vi "TCP-Com_StandAlone.vi"(8 "Exit Control Label":string="Exit Button", 9 "pwd":string, 10 "LabView Port":u16=4000, 11 "VI Refnum":refnum<vi>) -> (0 "error out":errorcluster)   [LabVIEW 2019]
doc: "This template is for the Queued Message Handler design pattern.\n\nThe Event Handling Loop generates messages based on user interface actions.\n\nThe Message Handling Loop processes messages generated by the Event Handling Loop, or by other messages. The messages are string values, so new messages can be added easily to the Message Cases case structure in the Message Handling Loop. Each message cluster can also provide an optional value for Message Data, which is a variant that can be converted to whatever message-specific data is required."
uses:
  support/TPC-Enum.ctl
  support/Global 1.vi
  support/Message Queue/Enqueue Message (Single).vi
  <vilib>/Utility/error.llb/Error Cluster From Error Code.vi
  <vilib>/ErrorRing/Error Ring.xnode
  support/Message Queue/Message Queue.lvlib
  support/User Event - Stop/User Event - Stop.lvlib
panel:
  out "Try reques  Bool":bool
  out "Sent to MIDAS":string
  out "connection ID":refnum<k5>
  out "Client Connected":bool
  in  "Request":string
  in  "Try request":bool
  in  "Exit":bool
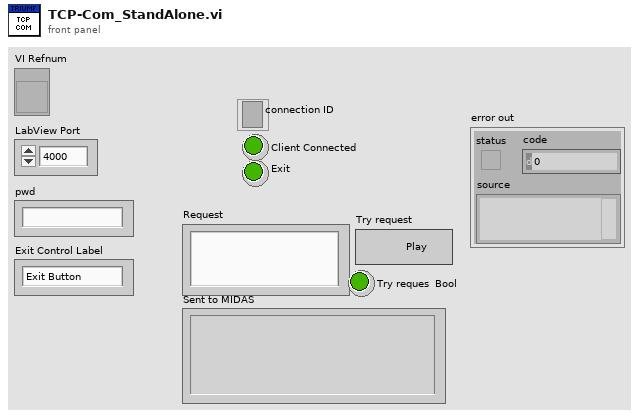
[diagram p1: front panel]
types:
  T1 = typedef "TPC-Enum.ctl" = enum16{"Wait For Client", "Check Client", "Listen"}
  T2 = typedef "Message Queue.lvlib/All Message Queues.ctl" = cluster{"TCP":refnum<queue>}
  T3 = enum16{"Standard", "Buffered", "CRLF", "Immediate"}
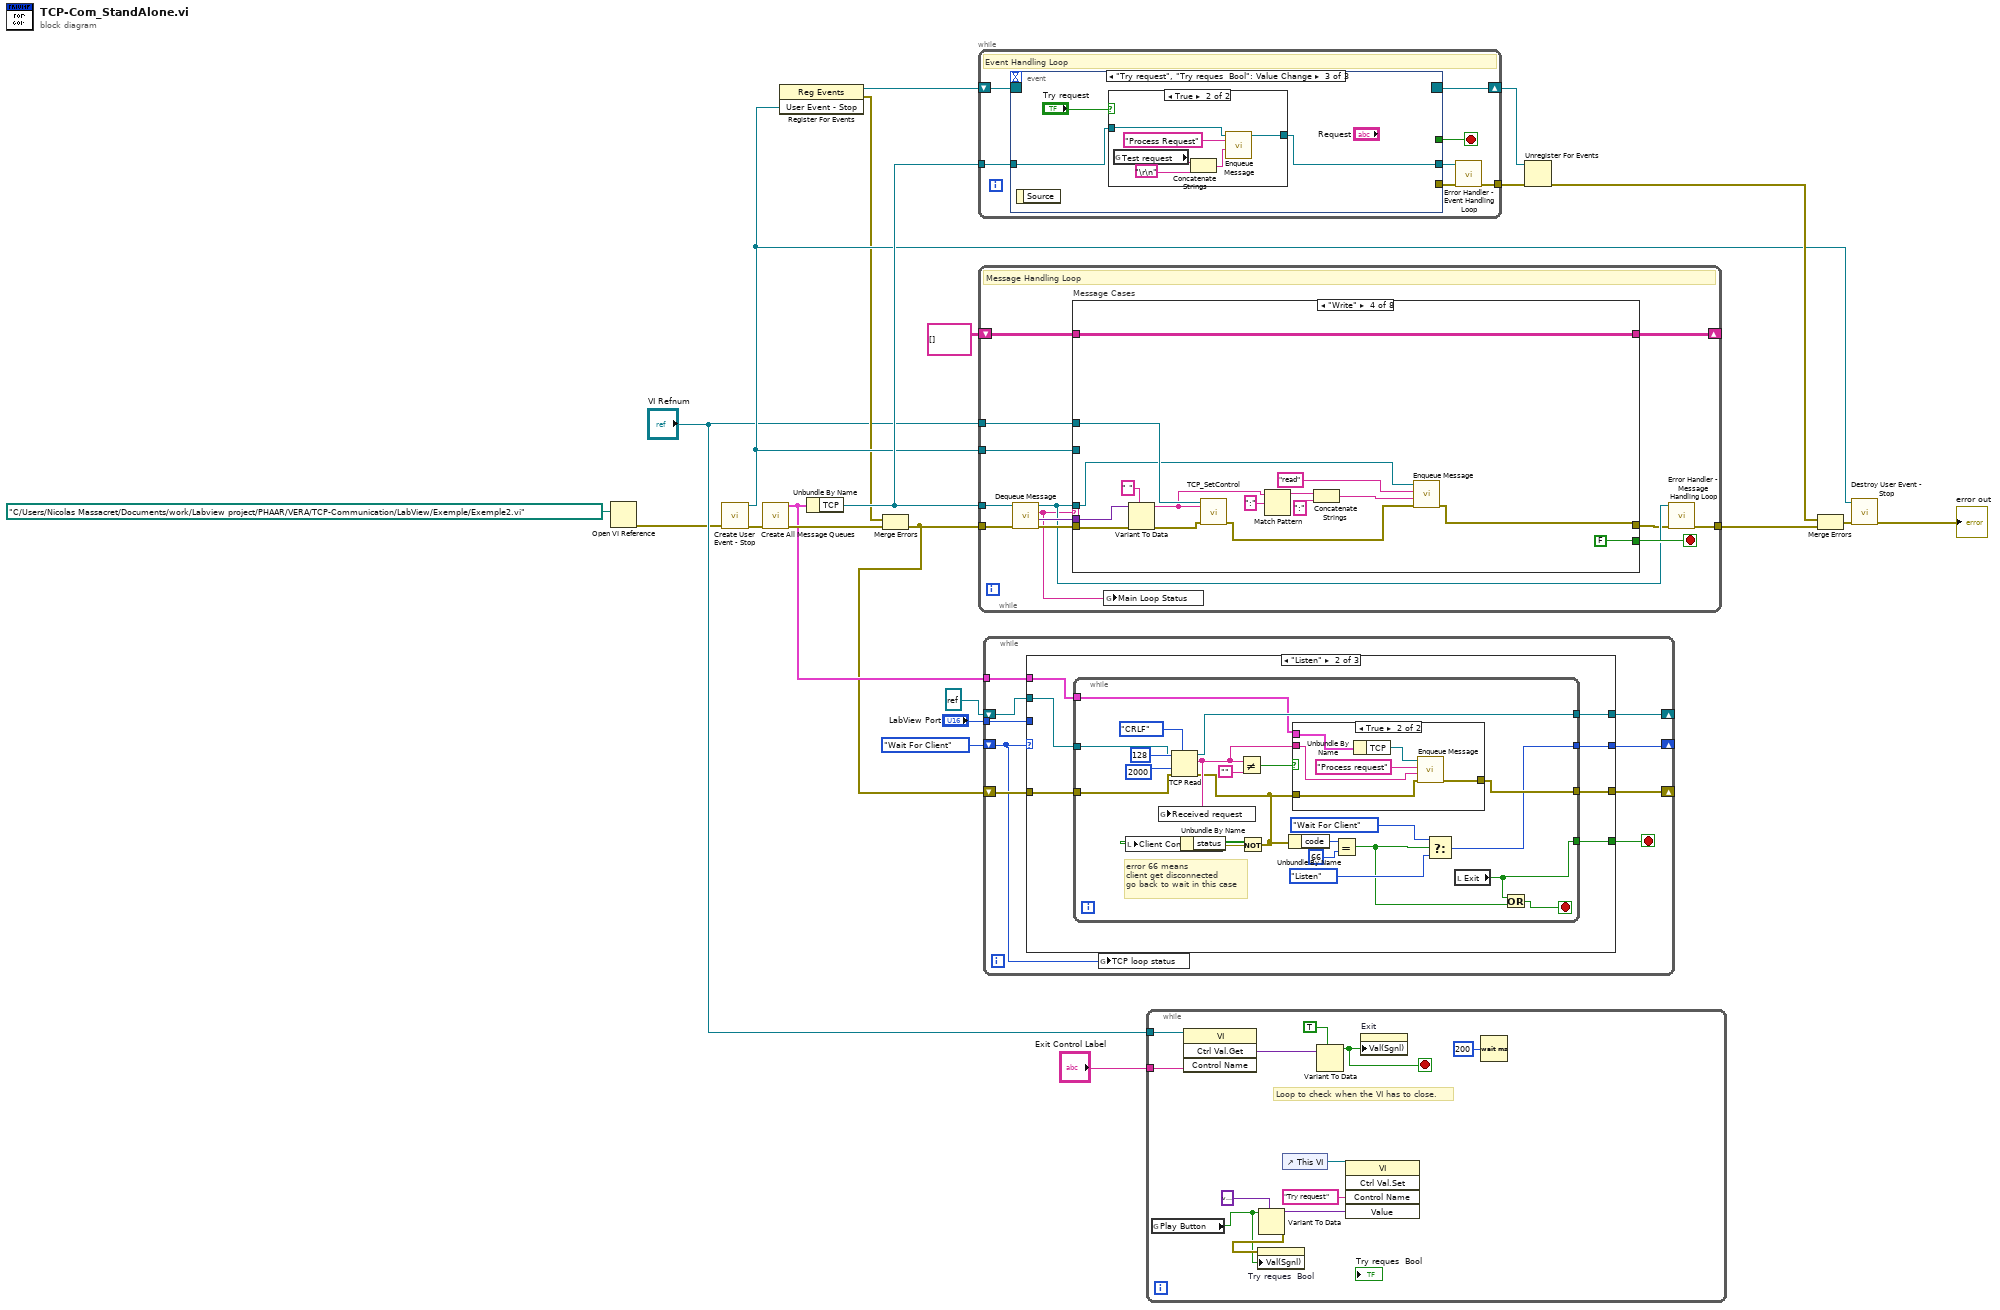
[diagram p0: block diagram]
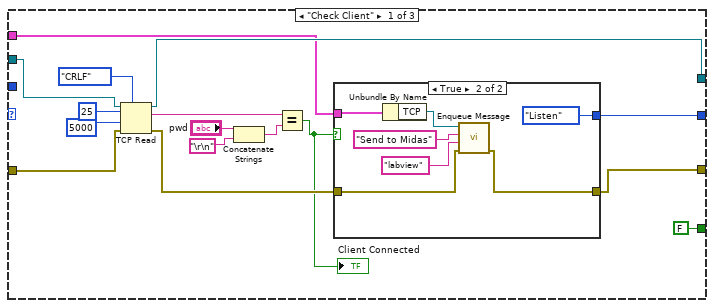
[diagram p2: hidden frame]
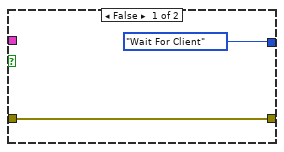
[diagram p3: hidden frame]
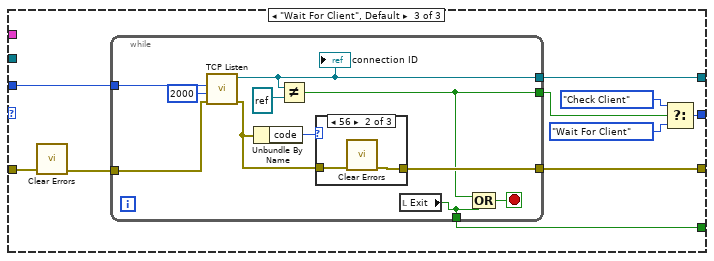
[diagram p5: hidden frame]
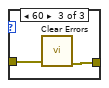
[diagram p7: hidden frame]
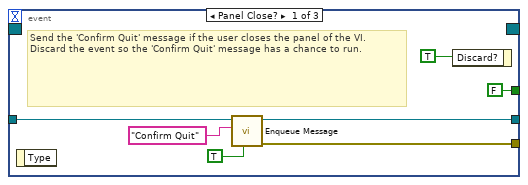
[diagram p8: hidden frame]
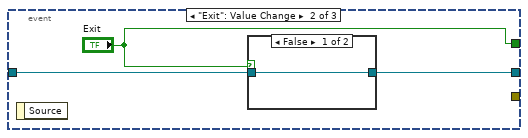
[diagram p9: hidden frame]
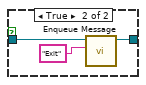
[diagram p10: hidden frame]
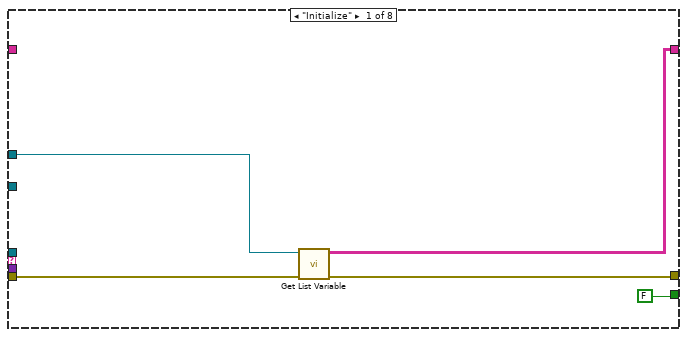
[diagram p12: hidden frame]
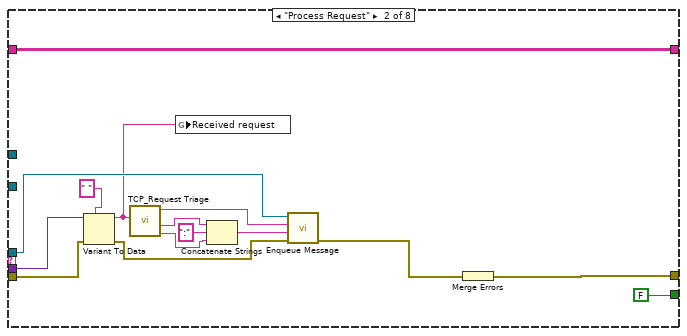
[diagram p13: hidden frame]
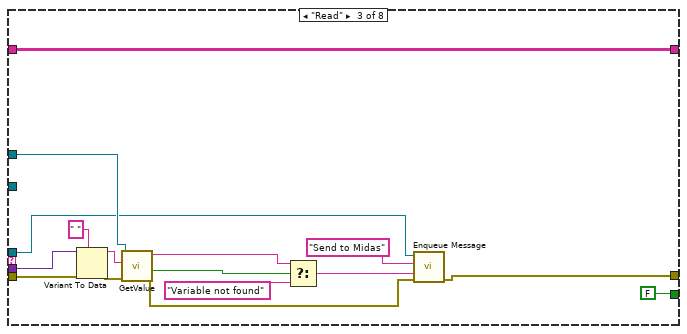
[diagram p14: hidden frame]
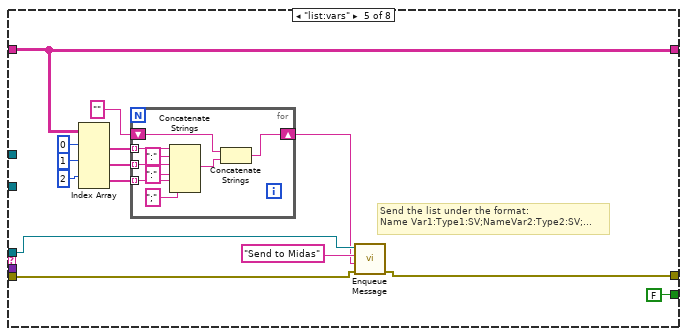
[diagram p15: hidden frame]
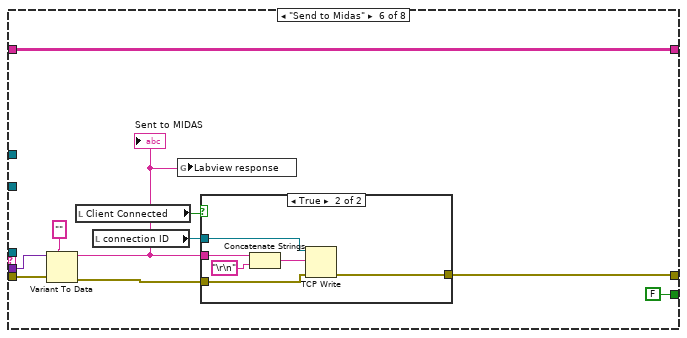
[diagram p16: hidden frame]
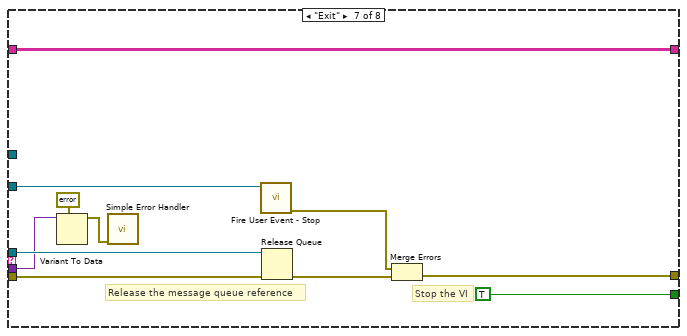
[diagram p18: hidden frame]
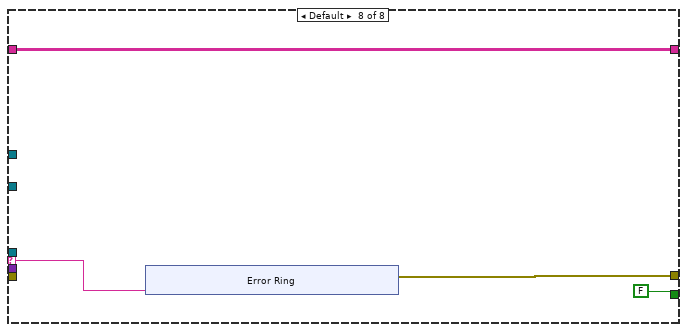
[diagram p19: hidden frame]
diagram:
  n1 = Open VI Reference(vi path=path "C:/Users/Nicolas Massacret/Documents/work/Labview project/PHAAR/VERA/TCP-Communication/LabView/Exemple/Exemple2.vi") -> (error out=w2:errorcluster)  [unwired: 5 in, 1 out]
  n2 = call "Create User Event - Stop.vi"("error in (no error)"=w2) -> ("error out"=w19:errorcluster, "User Event - Stop"=w13:refnum<user-event>)  [unwired: 9 in]
  n3 = call "Create All Message Queues.vi"("error in (no error)"=w19) -> ("error out"=w22:errorcluster, "Message Queues out"=w8:T2)  [unwired: 9 in]
  n4 = register-events(w13) -> (reference out=w14:refnum<event-registration>, error out=w12:errorcluster)  [unwired: 2 in]
  n5 = Unbundle By Name(w8) -> ("TCP"=w20:refnum<queue>)
  n6 = Merge Errors(w12, w22) -> (w4:errorcluster)
  n7 = while {
    tunnel: w20 -> [w29]
    shift-right: [w27] -> w16
    shift-left: w14 -> [w28]
    tunnel: [w23] -> w15
    stop <- w25 stop-if-true
    # "Event Handling Loop"
    n8 = event shown="[2] \"Try request\", \"Try reques  Bool\": Value Change" {
      selector: w28 -> [_ _ _]
      dyn-events: [_ _ _] -> w27
      timeout: _ -> [_ _ _]
      tunnel: [FALSE ("Discard?") "Exit" _] -> w25
      tunnel: w29 -> [w35 w39 w45]
      tunnel: [w34 _ _] -> w26
      tunnel: [w33 w38 w44] -> w24
      event Panel Close? {
        # "Send the 'Confirm Quit' message if the user closes the panel of the VI. Discard the event so the 'Confirm Quit' message has a chance to run."
        n9 = event-data() -> ()  [unwired: 1 in, 1 out]
        n10 = call-poly "Enqueue Message.vi"("Priority Message? (F)"=TRUE, "Message"="Confirm Quit", "Message Queue"=w35) -> ("error out"=w34:errorcluster, "dup Message Queue"=w33:refnum<queue>)  [unwired: 7 in]
        n11 = event-data("Discard?"=TRUE) -> ()  [unwired: 1 in, 1 out]
      }
      event "Exit": Value Change {
        n12 = event-data() -> ()  [unwired: 1 in, 1 out]
        n13 = case shown="False" "Exit" {
          tunnel: w39 -> [w40 w43]
          tunnel: [w40 w41] -> w38
          frame False {
          }
          frame True {
            n14 = call-poly "Enqueue Message.vi"("Message"="Exit", "Message Queue"=w43) -> ("dup Message Queue"=w41:refnum<queue>)  [unwired: 8 in, 1 out]
          }
        }
      }
      event "Try request", "Try reques  Bool": Value Change {
        n15 = event-data() -> ()  [unwired: 1 in, 1 out]
        n16 = case shown="True" "Try request" {
          tunnel: w45 -> [w47 w53]
          tunnel: [w47 w52] -> w44
          frame False {
          }
          frame True {
            n17 = global read "Global 1.vi" "Test request"() -> (w48:string)
            n18 = Concatenate Strings(w48, "\r\n") -> (w51:string)
            n19 = call-poly "Enqueue Message.vi"("Message Data"=w51, "Message"="Process Request", "Message Queue"=w53) -> ("dup Message Queue"=w52:refnum<queue>)  [unwired: 7 in, 1 out]
          }
        }
      }
    }
    n20 = call "Error Handler - Event Handling Loop.vi"("error in (no error)"=w26, "Message Queue"=w24) -> ("dup error in"=w23:errorcluster)  [unwired: 8 in, 1 out]
  }
  n21 = while {
    tunnel: w20 -> [w61]
    tunnel: w13 -> [w65]
    tunnel: w4 -> [w64]
    tunnel: [w59] -> w21
    tunnel: "VI Refnum" -> [w57]
    shift-right: [w56] -> _
    shift-left: string[][] [] -> [w55]
    stop <- w66 stop-if-true
    # "Message Handling Loop"
    n22 = call "Dequeue Message.vi"("error in (no error)"=w64, "Message Queue"=w61) -> ("error out"=w63:errorcluster, "Message Data"=w62:variant, "Message"=w54:string, "dup Message Queue"=w60:refnum<queue>)  [unwired: 6 in]
    n23 = case "Message Cases" shown="\"Write\"" w54 {
      selector: w54 -> [_ _ _ _ _ _ _ w172]
      tunnel: w60 -> [_ w79 w88 w105 w131 _ w169 _]
      tunnel: w63 -> [w70 w84 w101 w117 w130 w149 w163 _]
      tunnel: [w67 w86 w87 w103 w129 w143 w166 w173] -> w58
      tunnel: [FALSE FALSE FALSE FALSE FALSE FALSE TRUE FALSE] -> w66
      tunnel: w62 -> [_ w85 w102 w116 _ w148 w160 _]
      tunnel: w65 -> [_ _ _ _ _ _ w165 _]
      tunnel: w57 -> [w69 _ w95 w113 _ _ _ _]
      tunnel: [w68 w73 w98 w114 w127 w151 w159 w170] -> w56
      tunnel: w55 -> [_ w73 w98 w114 w127 w151 w159 w170]
      frame "Initialize" {
        # "Initialize - All initialization work should take place in this message, since other loops can potentially enqueue messages that execute immediately after this one."
        n24 = call "Get List Variable.vi"("error in (no error)"=w70, "VI in"=w69) -> ("error out"=w67:errorcluster, "Array"=w68:string[][])  [unwired: 8 in]
      }
      frame "Process Request" {
        # "Something - Replace this message with functionality for your own application."
        n25 = Variant To Data(error in=w84, type=" " ("Message"), Variant=w85) -> (data=w72:string, error out=w80:errorcluster)
        n26 = call "TCP_Request Triage.vi"("Message"=w72) -> ("Value"=w75:string, "Variable"=w76:string, "Request"=w77:string)  [unwired: 8 in]
        n27 = global write "Global 1.vi" "Received request"(w72) -> ()
        n28 = Concatenate Strings(w76, ":" ("string"), w75) -> (w78:string)
        n29 = call-poly "Enqueue Message.vi"("error in (no error)"=w80, "Message Data"=w78, "Message"=w77, "Message Queue"=w79) -> ("error out"=w81:errorcluster)  [unwired: 6 in, 1 out]
        n30 = Merge Errors(w81) -> (w86:errorcluster)
      }
      frame "Read" {
        n31 = Variant To Data(error in=w101, type=" " ("Message"), Variant=w102) -> (data=w96:string, error out=w97:errorcluster)
        n32 = call "GetValue.vi"("reference"=w95, "Input"=w96, "error in (no error)"=w97) -> ("Answer"=w92:string, "Found?"=w93:bool, "error out"=w91:errorcluster)  [unwired: 5 in]
        n33 = Select(t=w92, s=w93, f="Variable not found") -> (s? t:f=w89:string)
        n34 = call-poly "Enqueue Message.vi"("error in (no error)"=w91, "Message Data"=w89, "Message"="Send to Midas", "Message Queue"=w88) -> ("error out"=w87:errorcluster)  [unwired: 6 in, 1 out]
      }
      frame "Write" {
        n35 = Variant To Data(error in=w117, type=" " ("Message"), Variant=w116) -> (data=w108:string, error out=w112:errorcluster)
        n36 = call "TCP_SetControl.vi"("VI Refnum"=w113, "Input"=w108, "error in (no error)"=w112) -> ("error out"=w104:errorcluster)  [unwired: 6 in, 1 out]
        n37 = Match Pattern(string=w108, regular expression=":") -> (before substring=w106:string)  [unwired: 1 in, 3 out]
        n38 = Concatenate Strings(w106, ":" ("string")) -> (w110:string)
        n39 = call-poly "Enqueue Message.vi"("error in (no error)"=w104, "Message Data"=w110, "Message"="read", "Message Queue"=w105) -> ("error out"=w103:errorcluster)  [unwired: 6 in, 1 out]
      }
      frame "list:vars" {
        # "Send the list under the format:\nName Var1:Type1:SV;NameVar2:Type2:SV;..."
        n40 = Index Array(array=w127, index (row) #1=0 ("index (row)"), index (row) #2=1 ("index (row)"), index (row) #3=2 ("index (row)")) -> (element #1=w125:string[], element #2=w123:string[], element #3=w119:string[])  [unwired: 3 in]
        n41 = for {
          tunnel: w125 -> [w141] mode=indexing
          tunnel: w123 -> [w139] mode=indexing
          shift-right: [w135] -> w121
          shift-left: "" -> [w137]
          tunnel: w119 -> [w134] mode=indexing
          n42 = Concatenate Strings(w141, ":" ("string"), w139, ":" ("string"), w134, ";" ("string")) -> (w136:string)
          n43 = Concatenate Strings(w137, w136) -> (w135:string)
        }
        n44 = call-poly "Enqueue Message.vi"("error in (no error)"=w130, "Message Data"=w121, "Message"="Send to Midas", "Message Queue"=w131) -> ("error out"=w129:errorcluster)  [unwired: 6 in, 1 out]
      }
      frame "Send to Midas" {
        n45 = Variant To Data(error in=w149, type="", Variant=w148) -> (data=w142:string, error out=w144:errorcluster)
        "Sent to MIDAS" <- w142
        n46 = local read "Client Connected"() -> (w146:bool)
        n47 = local read "connection ID"() -> (w145:refnum<k5>)
        n48 = global write "Global 1.vi" "Labview response"(w142) -> ()
        n49 = case shown="True" w146 {
          tunnel: w145 -> [_ w155]
          tunnel: w142 -> [_ w158]
          tunnel: w144 -> [w152 w156]
          tunnel: [w152 w154] -> w143
          frame False {
          }
          frame True {
            n50 = Concatenate Strings(w158, "\r\n") -> (w153:string)
            n51 = TCP Write(connection ID=w155, data in=w153, error in (no error)=w156) -> (error out=w154:errorcluster)  [unwired: 1 in, 2 out]
          }
        }
      }
      frame "Exit" {
        # "Stop the VI"
        # "Release the message queue reference"
        # "Exit - Exit the application."
        n52 = Variant To Data(type=errorcluster {"status"=FALSE, "code"=0, "source"=""} ("error constant"), Variant=w160) -> (data=w161:errorcluster)  [unwired: 1 in, 1 out]
        n53 = call <vilib>:"Simple Error Handler.vi"("error in (no error)"=w161) -> ()  [unwired: 4 in, 5 out]
        n54 = call "Fire User Event - Stop.vi"("User Event - Stop"=w165) -> ("error out"=w164:errorcluster)  [unwired: 10 in]
        n55 = Release Queue(queue=w169, error in (no error)=w163) -> (error out=w167:errorcluster)  [unwired: 1 in, 2 out]
        n56 = Merge Errors(w164, w167) -> (w166:errorcluster)
      }
      frame Default {
        # "'Default' case only runs if there is a message that isn't defined in any of the other cases.  Output a programming error."
        n57 = xnode "Error Ring"("parameter 0"=w172) -> ("error out"=w173:errorcluster)
      }
    }
    n58 = global write "Global 1.vi" "Main Loop Status"(w54) -> ()
    n59 = call "Error Handler - Message Handling Loop.vi"("error in (no error)"=w58, "Message Queue"=w60) -> ("dup error in"=w59:errorcluster)  [unwired: 8 in, 1 out]
  }
  n60 = while {
    shift-right: [w187] -> _
    shift-left: TPC-Enum."Wait For Client" -> [w181]
    tunnel: "LabView Port" -> [w189]
    shift-right: [w188] -> _
    shift-left: refnum<k5> refnum ("connection ID") -> [w183]
    shift-right: [w186] -> _
    shift-left: w4 -> [w185]
    tunnel: w8 -> [w182]
    stop <- w184 stop-if-true
    n61 = case shown="\"Listen\"" w181 {
      tunnel: w189 -> [_ _ w260]
      tunnel: w185 -> [w202 w220 w252]
      tunnel: [w196 w219 w259] -> w188
      tunnel: [w193 w216 w255] -> w187
      tunnel: [FALSE w215 w254] -> w184
      tunnel: [w192 w217 w253] -> w186
      tunnel: w183 -> [w201 w221 _]
      tunnel: w182 -> [w195 w218 _]
      frame "Check Client" {
        n62 = TCP Read(connection ID=w201, bytes to read=25, error in (no error)=w202, 7:T3."CRLF" ("mode (standard)"), 9:5000 ("timeout ms (25000)")) -> (connection ID out=w196:refnum<k5>, data out=w198:string, error out=w194:errorcluster)
        n63 = Concatenate Strings("pwd", "\r\n") -> (w197:string)
        n64 = Equal?(x=w198, y=w197) -> (x = y?=w190:bool)
        "Client Connected" <- w190
        n65 = case shown="True" w190 {
          tunnel: w195 -> [_ w214]
          tunnel: w194 -> [w207 w210]
          tunnel: [TPC-Enum."Wait For Client" TPC-Enum."Listen"] -> w193
          tunnel: [w207 w208] -> w192
          frame False {
          }
          frame True {
            n66 = Unbundle By Name(w214) -> ("TCP"=w213:refnum<queue>)
            n67 = call-poly "Enqueue Message.vi"("error in (no error)"=w210, "Message Data"="labview", "Message"="Send to Midas", "Message Queue"=w213) -> ("error out"=w208:errorcluster)  [unwired: 6 in, 1 out]
          }
        }
      }
      frame "Listen" {
        n68 = while {
          tunnel: w221 -> [w240]
          tunnel: w220 -> [w239]
          tunnel: [w236] -> w219
          tunnel: w218 -> [w235]
          tunnel: [w234] -> w217
          tunnel: [w230] -> w216
          tunnel: [w224] -> w215
          stop <- w223 stop-if-true
          # "error 66 means\nclient get disconnected\ngo back to wait in this case"
          n69 = TCP Read(connection ID=w240, bytes to read=128, error in (no error)=w239, 7:T3."CRLF" ("mode (standard)"), 9:2000 ("timeout ms (25000)")) -> (connection ID out=w236:refnum<k5>, data out=w228:string, error out=w227:errorcluster)
          n70 = global write "Global 1.vi" "Received request"(w228) -> ()
          n71 = Unbundle By Name(w227) -> ("status"=w233:bool)
          n72 = Not Equal?(x=w228, y="") -> (x != y?=w237:bool)
          n73 = Not(x=w233) -> (.not. x?=w229:bool)
          n74 = local write "Client Connected"(w229) -> ()
          n75 = Unbundle By Name(w227) -> ("code"=w226:i32)
          n76 = case shown="True" w237 {
            tunnel: w228 -> [_ w247]
            tunnel: w235 -> [_ w248]
            tunnel: w227 -> [w244 w246]
            tunnel: [w244 w245] -> w234
            frame False {
            }
            frame True {
              n77 = Unbundle By Name(w248) -> ("TCP"=w250:refnum<queue>)
              n78 = call-poly "Enqueue Message.vi"("error in (no error)"=w246, "Message Data"=w247, "Message"="Process request", "Message Queue"=w250) -> ("error out"=w245:errorcluster)  [unwired: 6 in, 1 out]
            }
          }
          n79 = Equal?(x=w226, y=66) -> (x = y?=w222:bool)
          n80 = Select(t=TPC-Enum."Wait For Client", s=w222, f=TPC-Enum."Listen") -> (s? t:f=w230:T1)
          n81 = local read "Exit"() -> (w224:bool)
          n82 = Or(x=w224, y=w222) -> (x .or. y?=w223:bool)
        }
      }
      frame "Wait For Client", Default {
        n83 = call <vilib>:"Clear Errors.vi"("error in (no error)"=w252) -> ("error out"=w251:errorcluster)  [unwired: 5 in, 1 out]
        n84 = while {
          tunnel: w260 -> [w271]
          tunnel: w251 -> [w269]
          tunnel: [w262] -> w258
          tunnel: [w267] -> w259
          tunnel: [w264] -> w253
          tunnel: [w261] -> w254
          stop <- w263 stop-if-true
          n85 = call <vilib>:"TCP Listen.vi"("error in (no error)"=w269, "timeout ms (wait forever: -1)"=2000, "port"=w271) -> ("error out"=w265:errorcluster, "connection ID"=w267:refnum<k5>)  [unwired: 4 in, 3 out]
          "connection ID" <- w267
          n86 = Unbundle By Name(w265) -> ("code"=w266:i32)
          n87 = Not Equal?(x=w267, y=refnum<k5> refnum ("connection ID")) -> (x != y?=w262:bool)
          n88 = case shown="56" w266 {
            tunnel: w265 -> [w272 w274 w276]
            tunnel: [w272 w273 w275] -> w264
            frame 0, Default {
            }
            frame 56 {
              n89 = call <vilib>:"Clear Errors.vi"("error in (no error)"=w274) -> ("error out"=w273:errorcluster)  [unwired: 5 in, 1 out]
            }
            frame 60 {
              n90 = call <vilib>:"Clear Errors.vi"("error in (no error)"=w276) -> ("error out"=w275:errorcluster)  [unwired: 5 in, 1 out]
            }
          }
          n91 = local read "Exit"() -> (w261:bool)
          n92 = Compound Arithmetic op=OR(w262, w261) -> (w263:bool)
        }
        n93 = Select(t=TPC-Enum."Check Client", s=w258, f=TPC-Enum."Wait For Client") -> (s? t:f=w255:T1)
      }
    }
    n94 = global write "Global 1.vi" "TCP loop status"(w181) -> ()
  }
  n95 = while {
    tunnel: "VI Refnum" -> [w283]
    tunnel: "Exit Control Label" -> [w284]
    stop <- w286 stop-if-true
    # "Loop to check when the VI has to close."
    n96 = global read "Global 1.vi" "Play Button"() -> (w277:bool)
    n97 = invoke class="VI" method="Ctrl Val.Get"(reference=w283, "Control Name"=w284) -> ("Get Control Value Variant"=w285:variant)  [unwired: 2 in, 3 out]
    n98 = Variant To Data(type=variant ("Value (Signaling)"), Variant=w277) -> (data=w280:variant, error out=w278:errorcluster)  [unwired: 1 in]
    n99 = property on="Try reques  Bool" class="Bool (strict)"(error in=w278, "Val(Sgnl)"=w277) -> ()  [unwired: 1 in, 2 out]
    n100 = control-ref of="This VI"() -> (w281:refnum<vi>)
    n101 = Variant To Data(type=TRUE, Variant=w285) -> (data=w286:bool)  [unwired: 1 in, 1 out]
    n102 = invoke class="VI" method="Ctrl Val.Set"(reference=w281, "Control Name"="Try request", "Value"=w280) -> ()  [unwired: 2 in, 5 out]
    n103 = property on="Exit" class="Bool (strict)"("Val(Sgnl)"=w286) -> ()  [unwired: 2 in, 2 out]
    n104 = Wait (ms)(milliseconds to wait=u32 200) -> ()  [unwired: 1 out]
  }
  n105 = Unregister For Events(event registration refnum=w16, error in=w15) -> (error out=w17:errorcluster)
  n106 = Merge Errors(w17, w21) -> (w18:errorcluster)
  n107 = call "Destroy User Event - Stop.vi"("error in (no error)"=w18, "User Event - Stop"=w13) -> ("error out"=→"error out":errorcluster)  [unwired: 9 in]
